vi "Adapt To Type.vi"(6 "Nulls as Defaults (F)":bool, 7 "Type and Defaults":variant, 8 "error in":errorcluster, 11 "Variant in":variant) -> (0 "error out":errorcluster, 3 "Variant out":variant)   [LabVIEW 2020, in "JKI JSON Serialization.lvlib"]
doc: "Converts previously parsed JSON string to the type specified by <b>Type and Defaults</b>. For any cluster element in Type and Defaults, the value of the element in Type and Default is used if element with the same name is not present in the JSON String. If <b>Nulls as Defaults </b> is true, returns the default value as provided in Type and Defaults when null value is encountered in input data structure."
uses:
  JKI JSON Serialization.lvlib
  Deserializer/JSON Deserializer/JSON Deserializer.lvclass
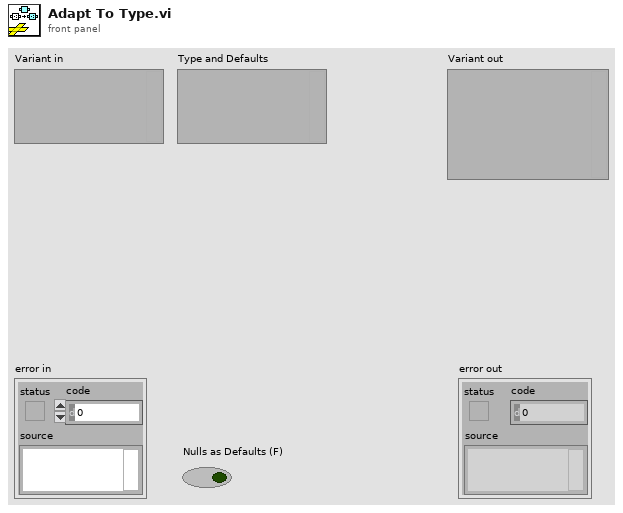
[diagram p1: front panel]
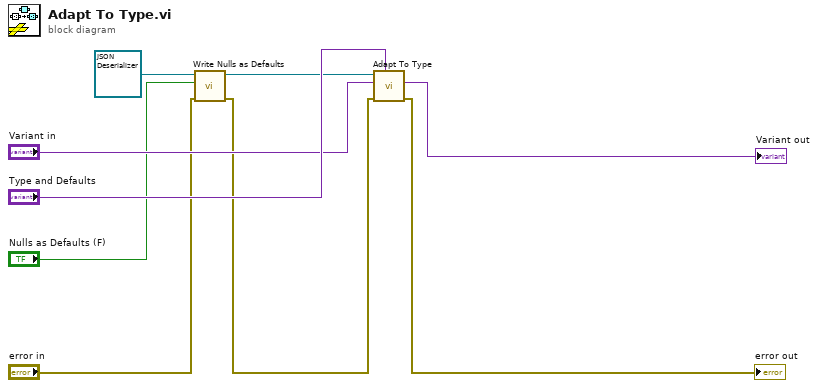
[diagram p0: block diagram]
diagram:
  n1 = call-dynamic "Write Nulls as Defaults.vi"("error in (no error)"="error in", "Nulls as Defaults"="Nulls as Defaults (F)", "JSON Deserializer in"=refnum<class "JSON Deserializer.lvclass"> refnum ("Deserializer in")) -> ("error out"=w2:errorcluster, "JSON Deserializer out"=w4:refnum<class "JSON Deserializer.lvclass">)  [unwired: 7 in]
  n2 = call-dynamic "Adapt To Type.vi"("Type and Defaults"="Type and Defaults", "error in (no error)"=w2, "Variant in"="Variant in", "Deserializer in"=w4) -> ("error out"=→"error out":errorcluster, "Variant out"=→"Variant out":variant)  [unwired: 5 in, 1 out]
